vi "Initialize.vi"(10 "Starting Month":u16(ring) items=["January", "February", "March", "April", "May", "June", "July", "August", "September", "October", "November", "December"]) -> (3 "Swapper For Priority Month":refnum<class "Swapper For Priority Month.lvclass">)   [LabVIEW 2023, in "Swapper For Priority Month.lvclass"]
uses:
  Swapper For Priority Month.lvclass
  Swapper For Priority Month.lvclass/Swapper For Priority Month.ctl
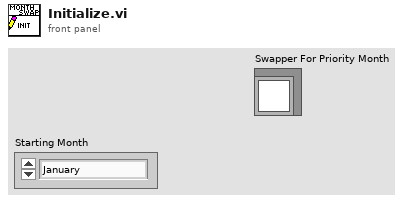
[diagram p1: front panel]
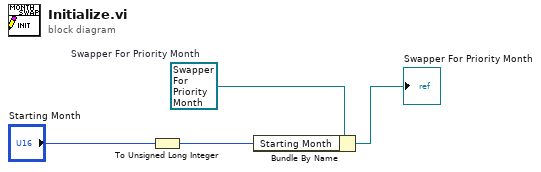
[diagram p0: block diagram]
diagram:
  w4 = refnum<class "Swapper For Priority Month.lvclass"> refnum  # Swapper For Priority Month
  n1 = To Unsigned Long Integer(number="Starting Month") -> (unsigned 32bit integer=w1:u32)
  n2 = Bundle By Name(cluster=w4, "Starting Month"=w1) -> (→"Swapper For Priority Month":refnum<class "Swapper For Priority Month.lvclass">)
